vi "insertGolden.vi"(6 "Station":string, 8 "error in (no error)":errorcluster, 9 "trans_time":string, 10 "machine":string, 11 "connection reference":T1) -> (0 "error out":errorcluster, 3 "connection reference 2":T1)   [LabVIEW 2012]
uses:
  <vilib>/addons/database/Connection.llb/Conn ObjectReference.ctl
  <vilib>/addons/database/Connection.llb/Conn Execute.vi
  <vilib>/addons/database/Recordset.llb/Rec Fetch Integer Data (R).vi
  <vilib>/addons/database/Recordset.llb/Rec Destroy - Connection.vi
  <vilib>/addons/database/NI_Database_API.lvlib
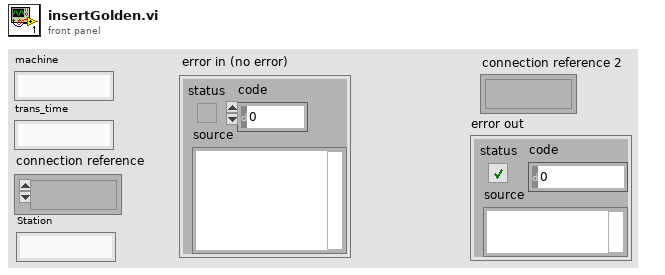
[diagram p1: front panel]
types:
  T1 = typedef "NI_Database_API.lvlib/Conn ObjectReference.ctl" = refnum<k1>
  T2 = typedef "NI_Database_API.lvlib/Rec ObjectReference.ctl" = refnum<k1>
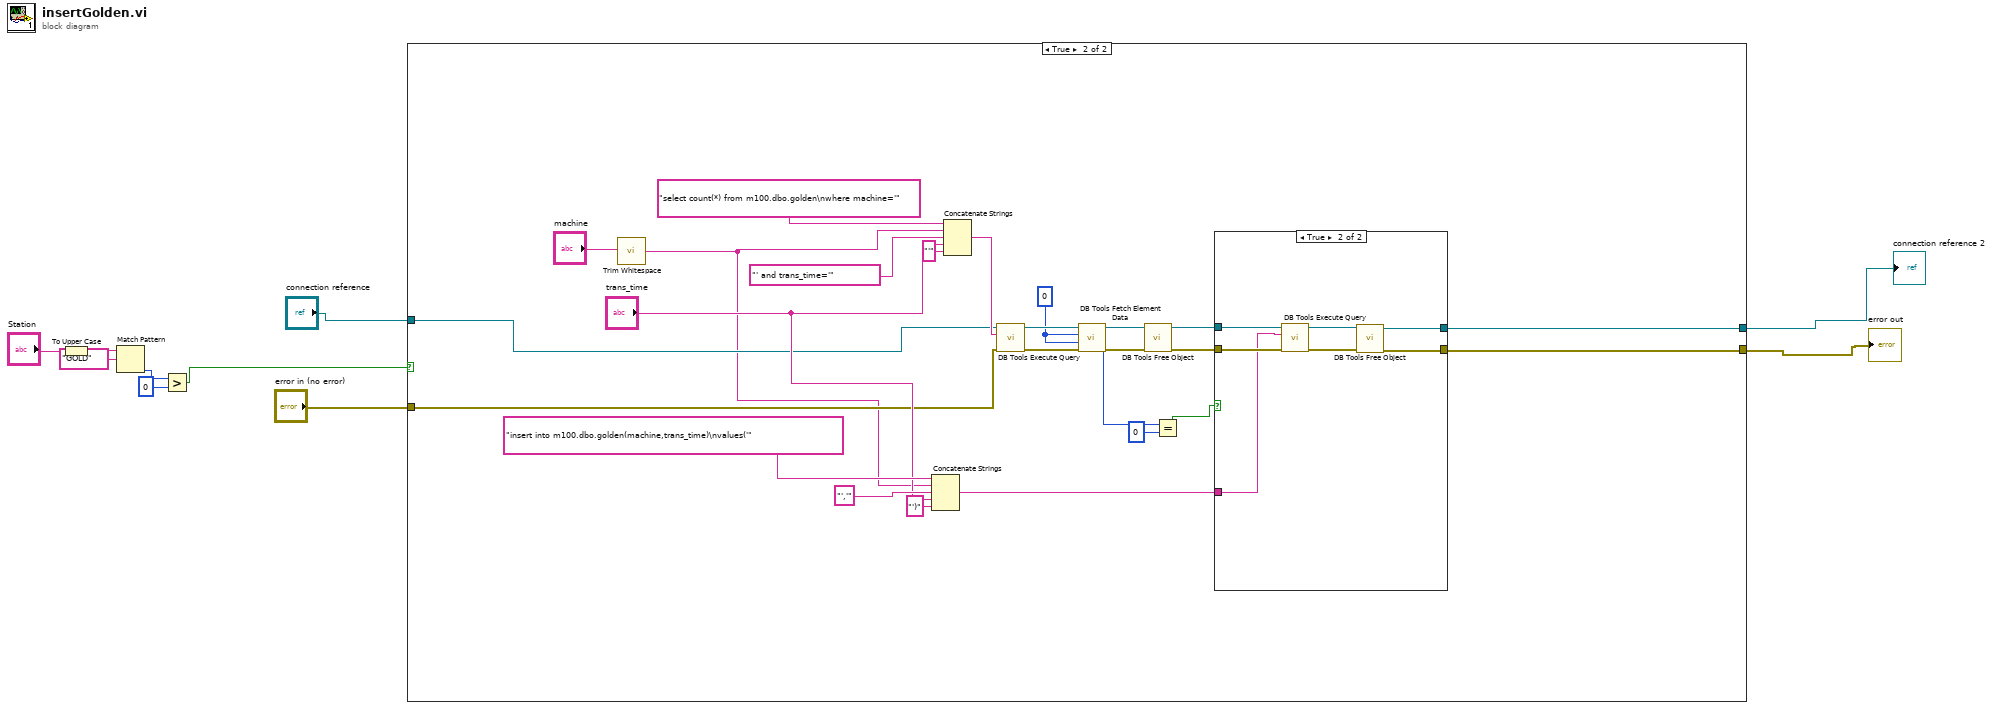
[diagram p0: block diagram]
diagram:
  n1 = To Upper Case(1:"Station") -> (0:w5:string)
  n2 = Match Pattern(string=w5, regular expression="GOLD") -> (offset past match=w3:i32)  [unwired: 1 in, 3 out]
  n3 = Greater?(x=w3, y=0) -> (0:w1:bool)
  n4 = case shown="True" w1 {
    tunnel: "connection reference" -> [w12 w18]
    tunnel: "error in (no error)" -> [w11 w17]
    tunnel: [w12 w16] -> w8
    tunnel: [w11 w15] -> w7
    frame False {
    }
    frame True {
      w29 = 0
      n5 = call <vilib>:"Trim Whitespace.vi"("string"="machine") -> ("trimmed string"=w13:string)  [unwired: 1 in]
      n6 = Concatenate Strings("insert into m100.dbo.golden(machine,trans_time)\nvalues('" ("string"), w13, "','" ("string"), "trans_time", "')" ("string")) -> (w19:string)
      n7 = Concatenate Strings("select count(*) from m100.dbo.golden\nwhere machine='" ("SQL query"), w13, "' and trans_time='" ("string"), "trans_time", "'" ("string")) -> (w30:string)
      n8 = call-poly <vilib>:"DB Tools Execute Query.vi"("error in (no error)"=w17, "SQL query"=w30, "connection reference"=w18) -> ("error out"=w35:errorcluster, "recordset reference"=w37:T2)  [unwired: 5 in]
      n9 = call-poly <vilib>:"DB Tools Fetch Element Data.vi"("error in (no error)"=w35, "type"=w29, "column index"=w29, "recordset reference"=w37) -> ("error out"=w34:errorcluster, "data"=w28:i32, "recordset reference out"=w36:T2)  [unwired: 3 in]
      n10 = call-poly <vilib>:"DB Tools Free Object.vi"("error in (no error)"=w34, "recordset reference"=w36) -> ("error out"=w24:errorcluster, "connection reference"=w25:T1)  [unwired: 8 in]
      n11 = Equal?(x=w28, y=0) -> (x = y?=w26:bool)
      n12 = case shown="True" w26 {
        tunnel: w25 -> [w39 w46]
        tunnel: w24 -> [w38 w45]
        tunnel: [w39 w43] -> w16
        tunnel: [w38 w41] -> w15
        tunnel: w19 -> [_ w40]
        frame False {
        }
        frame True {
          n13 = call-poly <vilib>:"DB Tools Execute Query.vi"("error in (no error)"=w45, "SQL query"=w40, "connection reference"=w46) -> ("error out"=w42:errorcluster, "recordset reference"=w44:T2)  [unwired: 5 in]
          n14 = call-poly <vilib>:"DB Tools Free Object.vi"("error in (no error)"=w42, "recordset reference"=w44) -> ("error out"=w41:errorcluster, "connection reference"=w43:T1)  [unwired: 8 in]
        }
      }
    }
  }
  "connection reference 2" <- w8
  "error out" <- w7
